vi "VPA QC LS and XDCR Zero.vi"(9 "DAQ Ref Cluster":T1, 10 "State Cluster":T3) -> (2 "State Cluster Out":T3)   [LabVIEW 2013]
uses:
  Controls/VPA QC State Data Cluster.ctl
  Controls/VPA QC General Cluster.ctl
  Controls/VPA QC State Enum.ctl
  Controls/VPA QC Bool Cluster.ctl
  Controls/VPA QC DAQ Ref Cluster.ctl
  Controls/VPA QC Scale Communication Settings DVR.ctl
  Controls/VPA QC Scale Communication Settings.ctl
panel:
  out "B side Low Warn":bool caption="Low Warning"
  out "A side Low Warn":bool caption="Low Warning"
  out "B side High Warn":bool caption="High Warning"
  out "A side High Warn":bool caption="High Warning"
  out "Quit":bool
  in  "Cancel":bool
  in  "Ok":bool
  out "B Reverse":bool
  out "B Forward":bool
  out "A Reverse":bool
  out "A Forward":bool
  out "_ZTB":dbl format="%#_5g"
  out "_ZTA":dbl format="%#_5g"
  # "Transducer and Limit Switch Tests"
  # "Ensure voltage of transducers are calibrated so they do not give negative numbers. Voltage can be adjusted by taking off the screw that is \nlabeled \"Zero\" and turning the screw. _ZTx values need to be higher than 100 but less than 200. Warning lights will show up for 2 seconds if\na value out of range is detected."
  # "Verify limit switch boards work by blacing a flag inplace of interruptors."
  # "Assembly Checklist"
  # "Assembly Checklist"
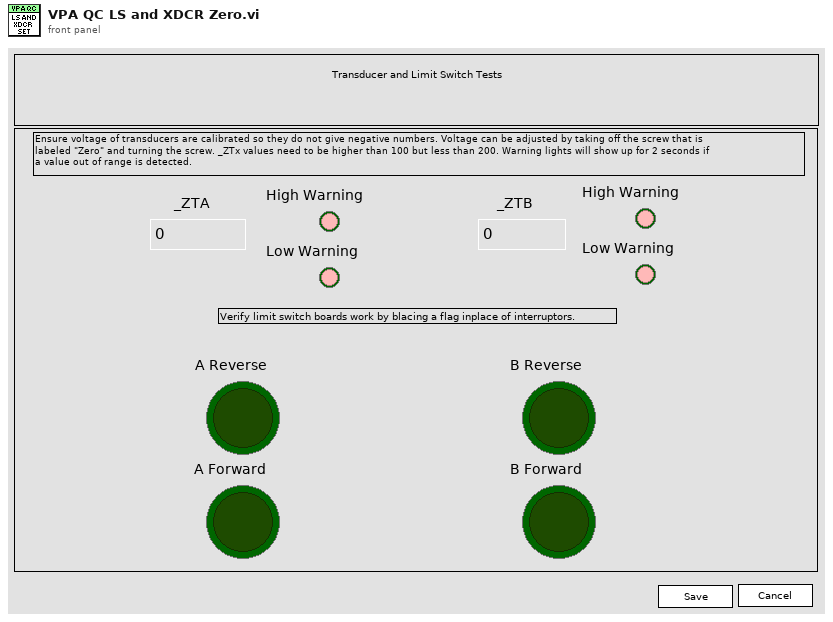
[diagram p1: front panel]
types:
  T1 = typedef "VPA QC DAQ Ref Cluster.ctl" = cluster{"IP Address of Pump":refnum<vi>, "Galil Ref":refnum<vi>, "VPA Connected?":refnum<vi>, "Pcur":refnum<vi>, "PcurA":refnum<vi>, "PcurB":refnum<vi>, "MLtot":refnum<vi>, "_LFA":refnum<vi>, "_LRA":refnum<vi>, "_LFB":refnum<vi>, "_LRB":refnum<vi>, "_ZTA":refnum<vi>, "_ZTB":refnum<vi>, "AI0 Volts":refnum<vi>, "AI1 Volts":refnum<vi>, "VPA Error":refnum<vi>, "Ain":refnum<vi>, "Aout":refnum<vi>, "Bin":refnum<vi>, "Bout":refnum<vi>, "Fstate":refnum<vi>, "XDCR 1\nOffset":refnum<vi>, "XDCR 2 \nOffset":refnum<vi>, "XDCR 1\nScale":refnum<vi>, "XDCR 2\nScale":refnum<vi>, "XDCR 1\nPSI":refnum<vi>, "XDCR 2\nPSI":refnum<vi>, "ReqStp":refnum<vi>, "Digital \nScale Read":refnum<vi>, "Scale Com\nSettings DVR":T2}
  T2 = typedef "VPA QC Scale Communication Settings DVR.ctl" = refnum<data-value>
  T3 = typedef "VPA QC State Data Cluster.ctl" = cluster{"XDCR 1":tag, "XDCR 2":tag, "General Information Clust":T4, "Assembly Checklist":cluster{"Ensure Drive Assembly checklist is completed.":bool, "Tighten Screws":bool, "Ensure VPA is wired correctly.":bool, "Ensure pump is running at voltage specified by customer.":bool}, "State":T5, "Manifold Leak Test Data":dbl[][], "Pressure Verification Test Data":dbl[][], "Flow Mode Verification Data":dbl[][], "DAQmx Error":errorcluster, "Bool Cluster":T6, "Leak Test Start Time":timestamp, "Pressure Test Start Time":timestamp, "Flow Test Start Time":timestamp, "Final Checklist cluster":cluster{"Check Fact Rest":bool, "Initialize Pump":bool, "Maintenance Hours":bool, "Clean Water Out":bool, "Covers":bool, "Screws":bool, "Wrap":bool, "Box":bool}, "Volts Constant":dbl, "Volume Constant A":dbl, "Volume Constant B":dbl, "Save File Path":path, "Comments Array":string[][], "File Format Version":u16}
  T4 = typedef "VPA QC General Cluster.ctl" = cluster{"Tech Name":string, "Date":timestamp, "Customer":string, "VPA Model":string, "G-72 Software Version":string, "Galil SN":string, "Galil Software Version":string, "VPA SN":string, "Valve SN":string, "Side A Drive Module SN":string, "Side B Drive Module SN":string, "A Side Transducer SN":string, "B Side Transducer SN":string, "A Side Motor SN":string, "B Side Motor SN":string, "A Side Gear Reducer SN":string, "B Side Gear Reducer SN":string, "A Side Limit Switch SN":string, "B Side Limit Switch SN":string, "Pump Voltage":string}
  T5 = typedef "VPA QC State Enum.ctl" = enum16{"General Information", "XDCR and LS Check", "Check Pump Function", "Manifold/Cylinder Leak Test", "Exit"}
  T6 = typedef "VPA QC Bool Cluster.ctl" = cluster{"Assembly":bool, "Gen":bool, "XDCR and LS Setup":bool, "Verify Pump Operation":bool, "Leak Test":bool, "Calibrate XDCRs":bool, "P Mode Verify":bool, "F Mode Verify":bool, "Vol Calibration":bool, "Flow Rate Test":bool, "Final Checklist":bool}
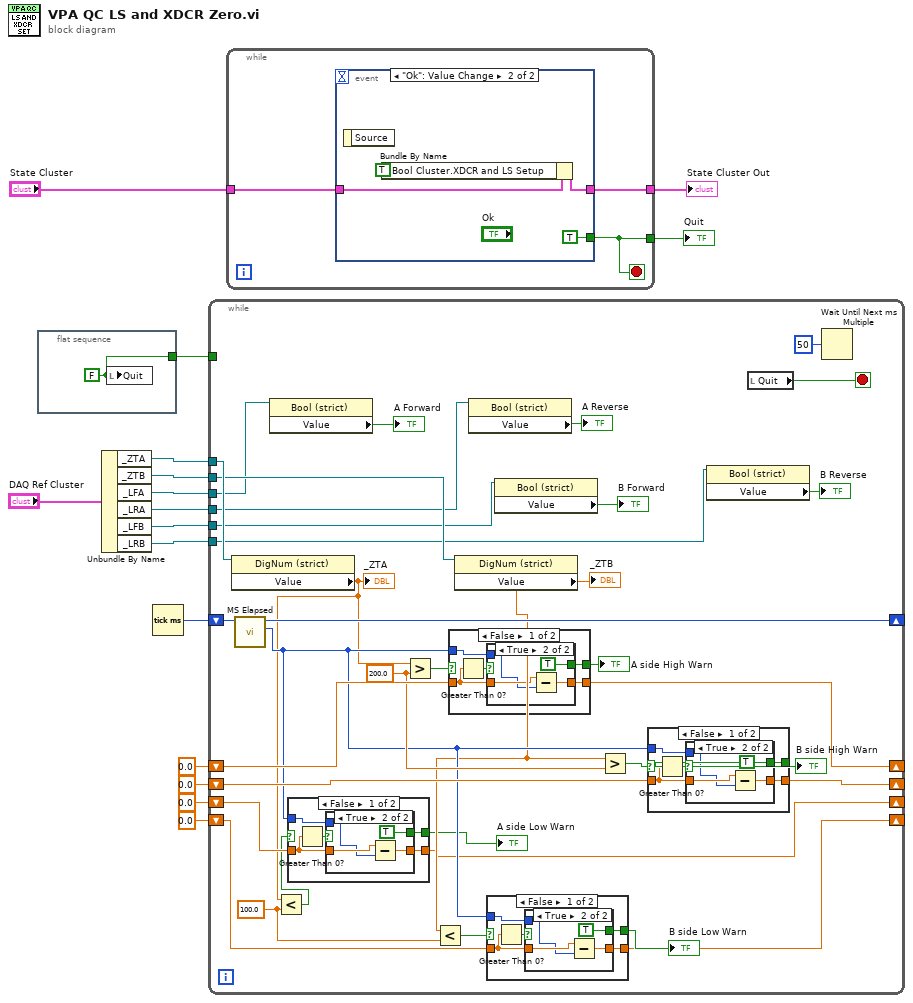
[diagram p0: block diagram]
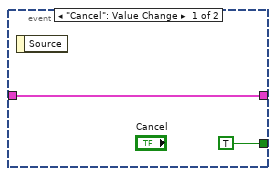
[diagram p2: hidden frame]
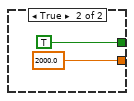
[diagram p4: hidden frame]
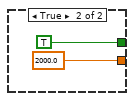
[diagram p6: hidden frame]
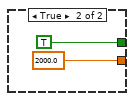
[diagram p8: hidden frame]
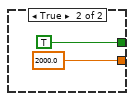
[diagram p10: hidden frame]
diagram:
  n1 = flat-sequence {
    tunnel: [w17] -> w8
    frame #0 {
      w17 = FALSE ("Quit")
      n2 = local write "Quit"(w17) -> ()
    }
  }
  n3 = Unbundle By Name("DAQ Ref Cluster") -> ("_ZTA"=w16:refnum<vi>, "_ZTB"=w15:refnum<vi>, "_LFA"=w14:refnum<vi>, "_LRA"=w13:refnum<vi>, "_LFB"=w12:refnum<vi>, "_LRB"=w11:refnum<vi>)
  n4 = Tick Count (ms)() -> (millisecond timer value=w3:u32)
  n5 = while {
    tunnel: w16 -> [w52]
    tunnel: w15 -> [w50]
    tunnel: w14 -> [w49]
    tunnel: w13 -> [w47]
    tunnel: w12 -> [w45]
    tunnel: w11 -> [w44]
    tunnel: w8 -> [_]
    shift-right: [w36] -> _
    shift-left: 0.0 ("ms in") -> [w37]
    shift-right: [w33] -> _
    shift-left: 0.0 ("ms in") -> [w34]
    shift-right: [w39] -> _
    shift-left: w3 -> [w40]
    shift-right: [w19] -> _
    shift-left: 0.0 ("ms in") -> [w28]
    shift-right: [w18] -> _
    shift-left: 0.0 ("ms in") -> [w27]
    stop <- w41 stop-if-true
    w23 = 100.0 ("y")
    w30 = 200.0 ("y")
    n6 = property class="DigNum (strict)"(reference=w52) -> ("Value"=w25:dbl)  [unwired: 1 in, 2 out]
    "_ZTA" <- w25
    n7 = call "MS Elapsed.vi"("ms in"=w40) -> ("elapsed ms"=w29:u32, "new ms time"=w39:u32)  [unwired: 9 in]
    n8 = property class="Bool (strict)"(reference=w49) -> ("Value"=→"A Forward":bool)  [unwired: 1 in, 2 out]
    n9 = Less?(x=w25, y=w23) -> (x < y?=w22:bool)
    n10 = case shown="False" w22 {
      tunnel: w28 -> [w68 _]
      tunnel: [w66 2000.0 ("ms in")] -> w19
      tunnel: [w65 TRUE] -> w21
      tunnel: w29 -> [w67 _]
      frame False {
        n11 = Greater Than 0?(x=w68) -> (x > 0?=w69:bool)
        n12 = case shown="True" w69 {
          tunnel: w68 -> [w70 w73]
          tunnel: w67 -> [_ w72]
          tunnel: [w70 w74] -> w66
          tunnel: [_ TRUE] -> w65
          frame False {
          }
          frame True {
            n13 = Subtract(x=w73, y=w72) -> (x-y=w74:dbl)
          }
        }
      }
      frame True {
      }
    }
    "A side Low Warn" <- w21
    n14 = Greater?(x=w25, y=w30) -> (0:w38:bool)
    n15 = case shown="False" w38 {
      tunnel: w37 -> [w92 _]
      tunnel: [w90 2000.0 ("ms in")] -> w36
      tunnel: [w89 TRUE] -> w35
      tunnel: w29 -> [w91 _]
      frame False {
        n16 = Greater Than 0?(x=w92) -> (x > 0?=w93:bool)
        n17 = case shown="True" w93 {
          tunnel: w92 -> [w94 w97]
          tunnel: w91 -> [_ w96]
          tunnel: [w94 w98] -> w90
          tunnel: [_ TRUE] -> w89
          frame False {
          }
          frame True {
            n18 = Subtract(x=w97, y=w96) -> (x-y=w98:dbl)
          }
        }
      }
      frame True {
      }
    }
    "A side High Warn" <- w35
    n19 = property class="DigNum (strict)"(reference=w50) -> ("Value"=w24:dbl)  [unwired: 1 in, 2 out]
    "_ZTB" <- w24
    n20 = Less?(x=w24, y=w23) -> (x < y?=w26:bool)
    n21 = property class="Bool (strict)"(reference=w47) -> ("Value"=→"A Reverse":bool)  [unwired: 1 in, 2 out]
    n22 = case shown="False" w26 {
      tunnel: w27 -> [w56 _]
      tunnel: [w54 2000.0 ("ms in")] -> w18
      tunnel: [w53 TRUE] -> w20
      tunnel: w29 -> [w55 _]
      frame False {
        n23 = Greater Than 0?(x=w56) -> (x > 0?=w57:bool)
        n24 = case shown="True" w57 {
          tunnel: w56 -> [w58 w61]
          tunnel: w55 -> [_ w60]
          tunnel: [w58 w62] -> w54
          tunnel: [_ TRUE] -> w53
          frame False {
          }
          frame True {
            n25 = Subtract(x=w61, y=w60) -> (x-y=w62:dbl)
          }
        }
      }
      frame True {
      }
    }
    "B side Low Warn" <- w20
    n26 = property class="Bool (strict)"(reference=w45) -> ("Value"=→"B Forward":bool)  [unwired: 1 in, 2 out]
    n27 = Greater?(x=w24, y=w30) -> (0:w31:bool)
    n28 = case shown="False" w31 {
      tunnel: w34 -> [w80 _]
      tunnel: [w78 2000.0 ("ms in")] -> w33
      tunnel: [w77 TRUE] -> w32
      tunnel: w29 -> [w79 _]
      frame False {
        n29 = Greater Than 0?(x=w80) -> (x > 0?=w81:bool)
        n30 = case shown="True" w81 {
          tunnel: w80 -> [w82 w85]
          tunnel: w79 -> [_ w84]
          tunnel: [w82 w86] -> w78
          tunnel: [_ TRUE] -> w77
          frame False {
          }
          frame True {
            n31 = Subtract(x=w85, y=w84) -> (x-y=w86:dbl)
          }
        }
      }
      frame True {
      }
    }
    "B side High Warn" <- w32
    n32 = property class="Bool (strict)"(reference=w44) -> ("Value"=→"B Reverse":bool)  [unwired: 1 in, 2 out]
    n33 = local read "Quit"() -> (w41:bool)
    n34 = Wait Until Next ms Multiple(millisecond multiple=u32 50) -> ()  [unwired: 1 out]
  }
  n35 = while {
    tunnel: "State Cluster" -> [w103]
    tunnel: [w102] -> w9
    tunnel: [w101] -> w7
    stop <- w101 stop-if-true
    n36 = event shown="[1] \"Ok\": Value Change" {
      selector: _ -> [_ _]
      dyn-events: _ -> [_ _]
      timeout: _ -> [_ _]
      tunnel: w103 -> [w105 w109]
      tunnel: [w105 w107] -> w102
      tunnel: [TRUE TRUE] -> w101
      event "Cancel": Value Change {
        n37 = event-data() -> ()  [unwired: 1 in, 1 out]
      }
      event "Ok": Value Change {
        n38 = event-data() -> ()  [unwired: 1 in, 1 out]
        n39 = Bundle By Name(cluster=w109, "Bool Cluster.XDCR and LS Setup"=TRUE ("Bool Cluster.XDCR 0 Adjust")) -> (w107:T3)
      }
    }
  }
  "State Cluster Out" <- w9
  "Quit" <- w7
